vi "Saturation Dequeue.vi"(8 "error in (no error)":errorcluster, 11 "Queue in":refnum<queue>) -> (0 "error out":errorcluster, 1 "Data":variant, 2 "State":T1, 3 "Queue out":refnum<queue>)   [LabVIEW 2017, in "Saturation.lvclass"]
uses:
  Saturation.lvclass
  Type Defs/Saturation State.ctl
  Expansion/Type Defs/Expansion State.ctl
  Saturation.lvclass/Saturation.ctl
  Expansion/Expansion.lvclass
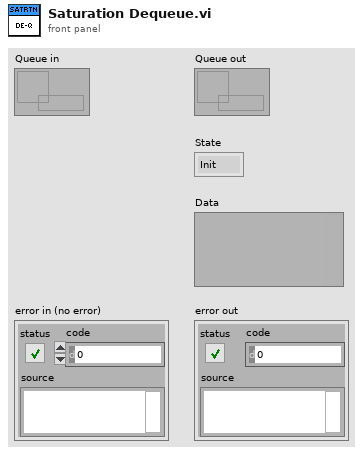
[diagram p1: front panel]
types:
  T1 = typedef "Saturation.lvclass/Saturation State.ctl" = enum16{"Init", "Go", "Stop", "Idle", "Error", "Shutdown"}
  T2 = typedef "Expansion.lvclass/Expansion State.ctl" = enum16{"Init", "Go", "Stop", "Idle", "Error", "Shutdown"}
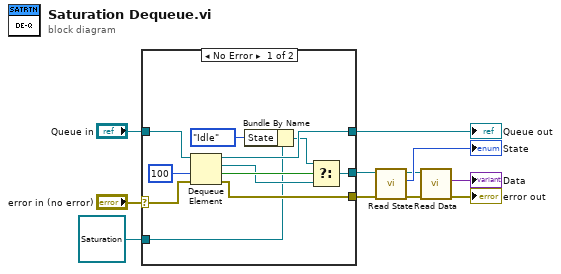
[diagram p0: block diagram]
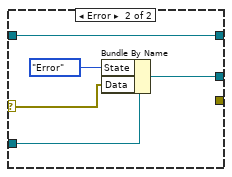
[diagram p2: hidden frame]
diagram:
  n1 = case shown="No Error" "error in (no error)" {
    selector: "error in (no error)" -> [w21 w24]
    tunnel: "Queue in" -> [w22 w27]
    tunnel: [w15 w26] -> w2
    tunnel: [w20 w27] -> w3
    tunnel: [w19 _] -> w1
    tunnel: refnum<class "Saturation.lvclass"> refnum ("Expansion.lvclass") -> [w12 w23]
    frame No Error {
      n2 = Dequeue Element(queue=w22, timeout in ms (-1)=100, error in (no error)=w21) -> (queue out=w20:refnum<queue>, element=w16:refnum<class "Saturation.lvclass">, timed out?=w17:bool, error out=w19:errorcluster)
      n3 = Bundle By Name(cluster=w12, "State"=Expansion_State."Idle") -> (w14:refnum<class "Saturation.lvclass">)
      n4 = Select(t=w14, s=w17, f=w16) -> (s? t:f=w15:refnum<class "Saturation.lvclass">)
    }
    frame Error {
      n5 = Bundle By Name(cluster=w23, "State"=Expansion_State."Error", "Data"=w24) -> (w26:refnum<class "Saturation.lvclass">)
    }
  }
  "Queue out" <- w3
  n6 = call "Read State.vi"("error in (no error)"=w1, "Expansion in"=w2) -> ("error out"=w8:errorcluster, "State"=→"State":T1, "Expansion out"=w10:refnum<class "Saturation.lvclass">)  [unwired: 7 in]
  n7 = call "Read Data.vi"("error in (no error)"=w8, "Expansion in"=w10) -> ("error out"=→"error out":errorcluster, "Data"=→"Data":variant)  [unwired: 7 in, 1 out]
